vi "joystick+grsim.vi"() -> ()   [LabVIEW 2016]
uses:
  <vilib>/Utility/inputDevices.llb/closeJoystick.vi
panel:
  out "error out":errorcluster
  out "port":u16
  in  "isteamyellow":bool=TRUE
  in  "Port:":u16=10020
  in  "SSL Vision Address:":string="224.5.23.2"
  out "16bit integer 3":i16
  out "16bit integer 2":i16
  out "16bit integer":i16
  out "appended array":u8[](array[numeric])
  out "error out 3":errorcluster
  in  "stop":bool
  in  "pos 1":i16=3468
  in  "pos 2":i16=3468
  in  "pos 3":i16=3468
  out "vel radial":u8[](array[numeric])
  out "vel normal":u8[](array[numeric])
  out "vel rotation":u8[](array[numeric])
  out "drible":u8
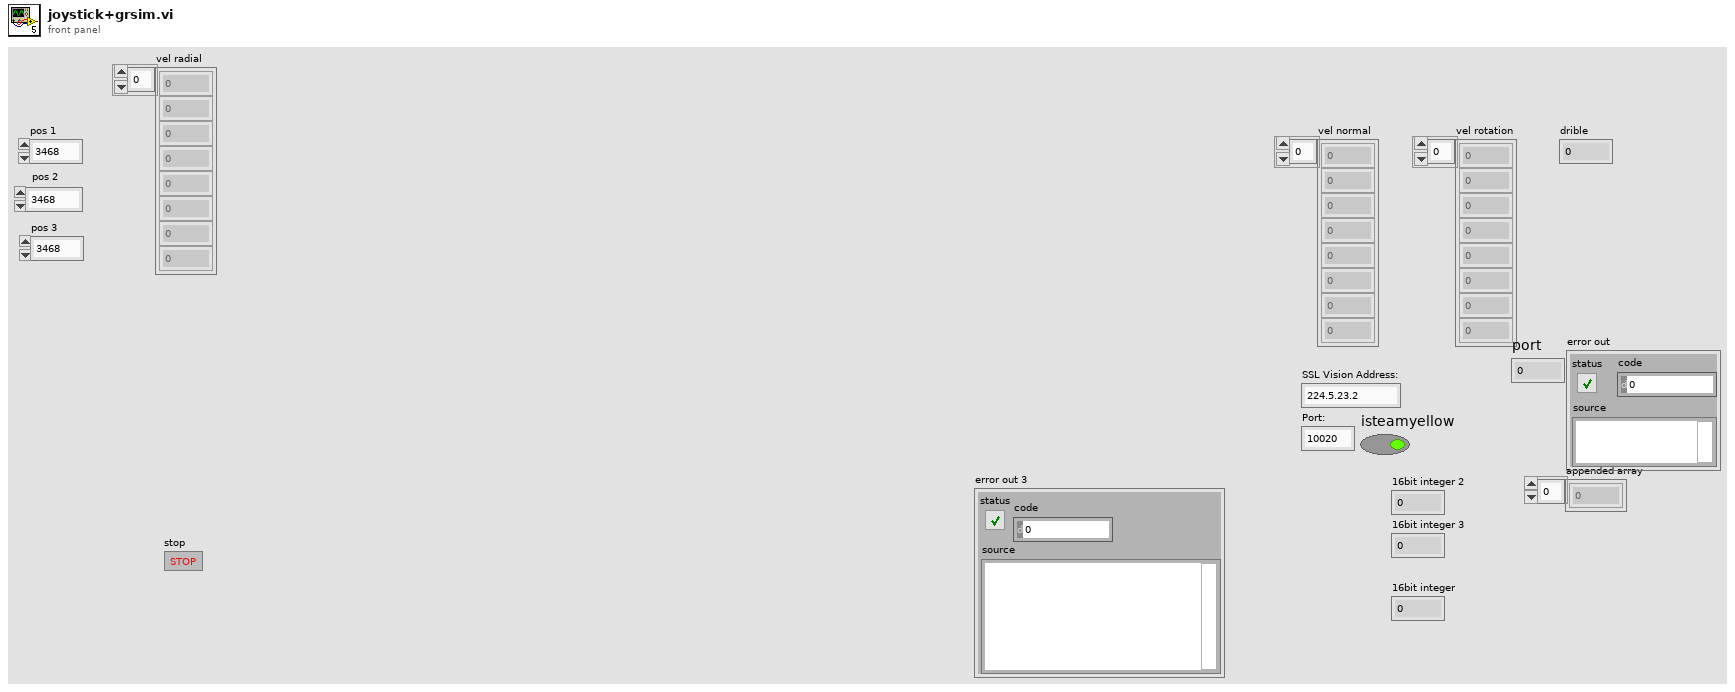
[diagram p1: front panel]
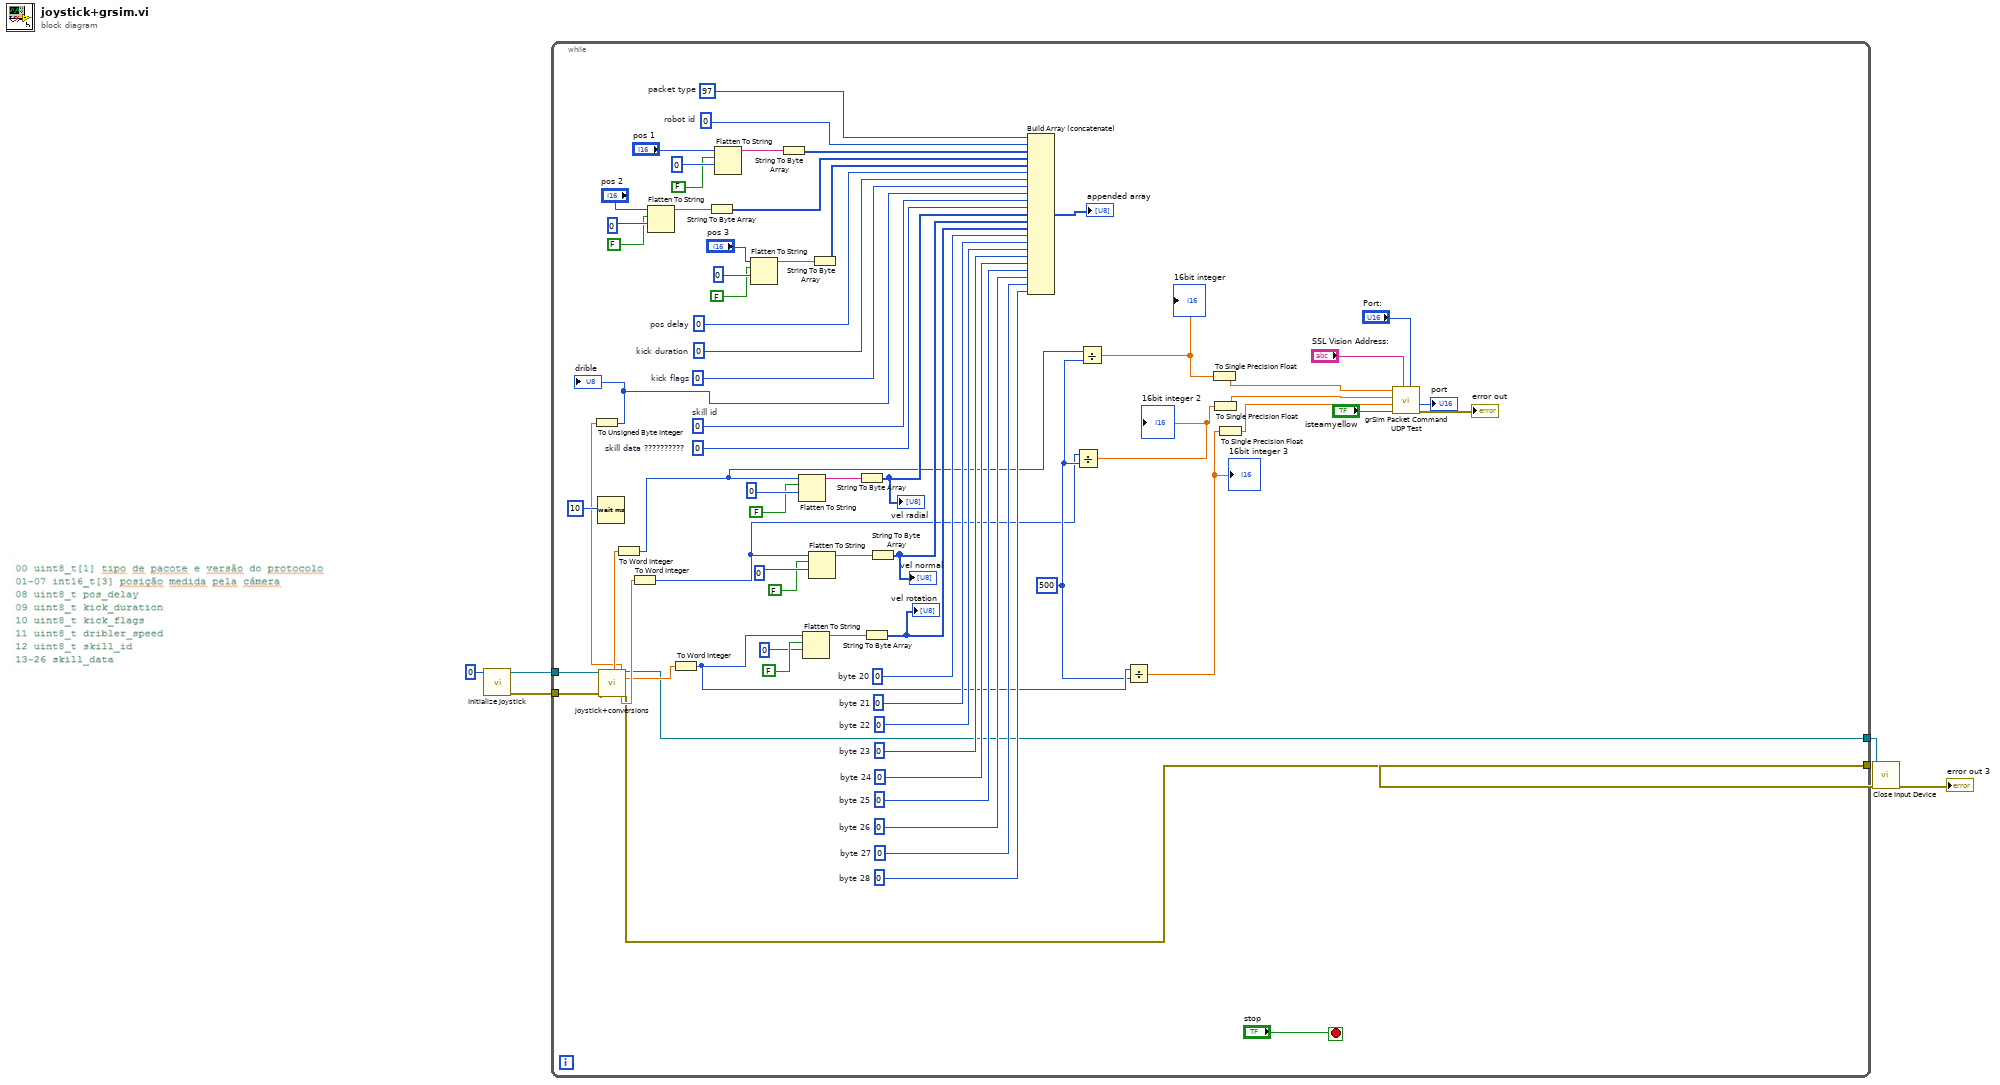
[diagram p0: block diagram]
diagram:
  n1 = call <vilib>:"Initialize Joystick.vi"("device index"=0) -> ("error out"=w4:errorcluster, "device ID"=w5:refnum<k1>)  [unwired: 9 in]
  n2 = while {
    tunnel: w5 -> [w33]
    tunnel: w4 -> [w32]
    tunnel: [w26] -> w2
    tunnel: [w25] -> w1
    stop <- "stop" stop-if-true
    w17 = 500
    w75 = u8 0  # skill data ??????????
    w72 = u8 0  # byte 28
    w71 = u8 0  # byte 27
    w70 = u8 0  # byte 26
    w68 = u8 0  # byte 25
    w69 = u8 0  # byte 24
    w67 = u8 0  # byte 23
    w66 = u8 0  # byte 22
    w65 = u8 0  # byte 21
    w64 = u8 0  # byte 20
    w58 = u8 0  # skill id
    w63 = u8 0  # kick flags
    w57 = u8 0  # kick duration
    w56 = u8 0  # pos delay
    w61 = u8 0  # robot id
    w34 = u8 97  # packet type
    n3 = Wait (ms)(milliseconds to wait=u32 10) -> ()  [unwired: 1 out]
    n4 = call "joystick+conversions.vi"("Refnum in"=w33, "error in (no error)"=w32) -> ("v_radial"=w31:dbl, "drible"=w27:dbl, "v_normal"=w30:dbl, "Refnum out"=w25:refnum<k1>, "R*w"=w29:dbl, "error out"=w26:errorcluster)  [unwired: 9 in, 11 out]
    n5 = To Unsigned Byte Integer(number=w27) -> (unsigned 8bit integer=w28:u8)
    "drible" <- w28
    n6 = To Word Integer(number=w31) -> (16bit integer=w19:i16)
    n7 = To Word Integer(number=w30) -> (16bit integer=w15:i16)
    n8 = Flatten To String(anything="pos 2", prepend array or string size? (T)=FALSE, byte order (0:big-endian, network order)=u16 0) -> (data string=w42:string)  [unwired: 1 in, 2 out]
    n9 = To Word Integer(number=w29) -> (16bit integer=w18:i16)
    n10 = String To Byte Array(string=w42) -> (unsigned byte array=w62:u8[])
    n11 = Flatten To String(anything="pos 1", prepend array or string size? (T)=FALSE, byte order (0:big-endian, network order)=u16 0) -> (data string=w37:string)  [unwired: 1 in, 2 out]
    n12 = Flatten To String(anything="pos 3", prepend array or string size? (T)=FALSE, byte order (0:big-endian, network order)=u16 0) -> (data string=w46:string)  [unwired: 1 in, 2 out]
    n13 = String To Byte Array(string=w37) -> (unsigned byte array=w38:u8[])
    n14 = Flatten To String(anything=w19, prepend array or string size? (T)=FALSE, byte order (0:big-endian, network order)=u16 0) -> (data string=w51:string)  [unwired: 1 in, 2 out]
    n15 = Flatten To String(anything=w18, prepend array or string size? (T)=FALSE, byte order (0:big-endian, network order)=u16 0) -> (data string=w55:string)  [unwired: 1 in, 2 out]
    n16 = Flatten To String(anything=w15, prepend array or string size? (T)=FALSE, byte order (0:big-endian, network order)=u16 0) -> (data string=w54:string)  [unwired: 1 in, 2 out]
    n17 = String To Byte Array(string=w46) -> (unsigned byte array=w48:u8[])
    n18 = String To Byte Array(string=w51) -> (unsigned byte array=w73:u8[])
    "vel radial" <- w73
    n19 = String To Byte Array(string=w55) -> (unsigned byte array=w74:u8[])
    "vel rotation" <- w74
    n20 = String To Byte Array(string=w54) -> (unsigned byte array=w22:u8[])
    "vel normal" <- w22
    n21 = Build Array (concatenate)(w34, w61, w38, w62, w48, w56, w57, w63, w28, w58, w75, w73, w22, w74, w64, w65, w66, w67, w69, w68, w70, w71, w72) -> (→"appended array":u8[])
    n22 = Divide(x=w15, y=w17) -> (x/y=w14:dbl)
    "16bit integer 2" <- w14
    n23 = Divide(x=w19, y=w17) -> (x/y=w16:dbl)
    "16bit integer" <- w16
    n24 = Divide(x=w18, y=w17) -> (x/y=w13:dbl)
    "16bit integer 3" <- w13
    n25 = To Single Precision Float(number=w16) -> (single precision float=w21:sgl)
    n26 = To Single Precision Float(number=w14) -> (single precision float=w20:sgl)
    n27 = To Single Precision Float(number=w13) -> (single precision float=w12:sgl)
    n28 = call "grSim Packet Command UDP Test.vi"("Port:"="Port:", "SSL Vision Address:"="SSL Vision Address:", "isteamyellow"="isteamyellow", "velangular"=w12, "velnormal"=w20, "veltangent"=w21) -> ("error out"=→"error out":errorcluster, "port"=→"port":u16)  [unwired: 4 in]
  }
  n29 = call-poly <vilib>:"Close Input Device.vi"("error in (no error)"=w2, "device ID"=w1) -> ("error out"=→"error out 3":errorcluster)  [unwired: 8 in]
